vi "Set_PowerHist_Range.vi"(7 "Slide":cluster{dbl, dbl}, 9 "View Subset":bool, 10 "Slide Ref":refnum<vi>, 11 "ChartRef":refnum<vi>) -> ()   [LabVIEW 2018]
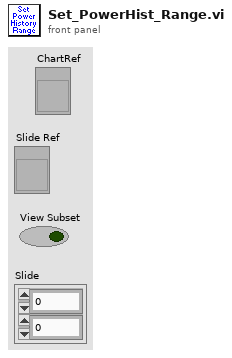
[diagram p1: front panel]
types:
  T1 = cluster{"Cal":dbl, "Cal Smooth":dbl, "Beac":dbl, "Beac Smooth":dbl, "NoiseFloorSum":dbl, "NoiseFloorSum Smooth":dbl}[]
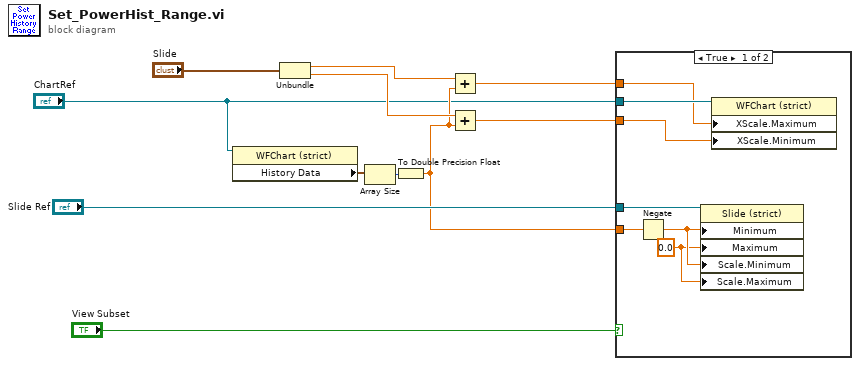
[diagram p0: block diagram]
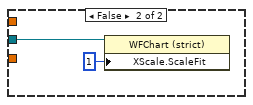
[diagram p2: hidden frame]
diagram:
  n1 = property class="WFChart (strict)"(reference="ChartRef") -> ("History Data"=w3:T1)  [unwired: 1 in, 2 out]
  n2 = Unbundle("Slide") -> (w9:dbl, w11:dbl)
  n3 = Array Size(array=w3) -> (size(s)=w4:i32)
  n4 = To Double Precision Float(number=w4) -> (double precision float=w7:dbl)
  n5 = Add(x=w9, y=w7) -> (x+y=w5:dbl)
  n6 = Add(x=w11, y=w7) -> (x+y=w6:dbl)
  n7 = case shown="True" "View Subset" {
    tunnel: "ChartRef" -> [w18 w20]
    tunnel: w5 -> [w17 _]
    tunnel: w6 -> [w16 _]
    tunnel: w7 -> [w14 _]
    tunnel: "Slide Ref" -> [w13 _]
    frame True {
      w12 = 0.0 ("Data Entry Limits:Maximum")
      n8 = Negate(x=w14) -> (-x=w15:dbl)
      n9 = property on="Property Node" class="Slide (strict)"(reference=w13, "Minimum"=w15, "Maximum"=w12, "Scale.Minimum"=w15, "Scale.Maximum"=w12) -> ()  [unwired: 1 in, 2 out]
      n10 = property class="WFChart (strict)"(reference=w18, "XScale.Maximum"=w17, "XScale.Minimum"=w16) -> ()  [unwired: 1 in, 2 out]
    }
    frame False {
      n11 = property class="WFChart (strict)"(reference=w20, "XScale.ScaleFit"=u8 1 ("X Scale.Scale Fit")) -> ()  [unwired: 1 in, 2 out]
    }
  }
